vi "RegisterTrends.vi"(8 "error in (no error)":errorcluster, 9 "asset node id":string, 10 "data group":string, 11 "data group map":variant) -> (0 "error out":errorcluster, 3 "data group map":variant)   [LabVIEW 2017, in "ModbusMaster.lvlib"]
uses:
  <vilib>/addons/InsightCM/Devices/Shared/Common/ModbusMaster/ModbusMaster.lvlib
  <vilib>/addons/InsightCM/Devices/Shared/Common/DataEventCreator/controls/Registry_Trend.ctl
  <vilib>/addons/InsightCM/Devices/Shared/Common/DataEventCreator/DataEventCreator.lvlib
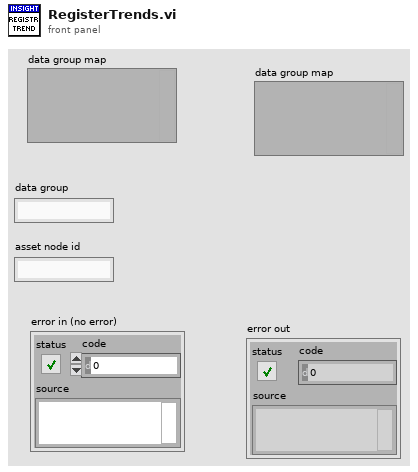
[diagram p1: front panel]
types:
  T1 = typedef "DataEventCreator.lvlib/Registry_Trend.ctl" = cluster{"TrendPointId":string, "DataSetName":string, "HighRate":bool, "Always Send":bool}
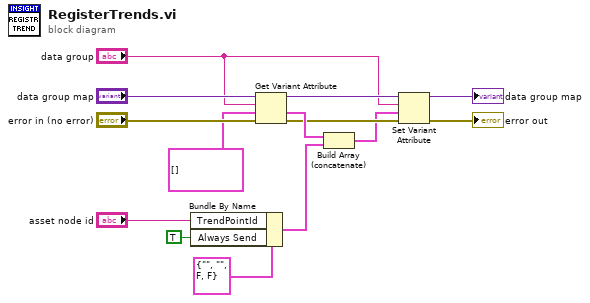
[diagram p0: block diagram]
diagram:
  n1 = Bundle By Name(cluster=T1 {"TrendPointId"="", "DataSetName"="", "HighRate"=FALSE, "Always Send"=FALSE} ("Trend"), "TrendPointId"="asset node id", "Always Send"=TRUE ("HighRate")) -> (w8:T1)
  n2 = Get Variant Attribute(Variant="data group map", name="data group", default value (empty Variant)=T1[] [], error in="error in (no error)") -> (duplicate Variant=w6:variant, value=w9:T1[], error out=w7:errorcluster)  [unwired: 1 out]
  n3 = Build Array (concatenate)(w9, w8) -> (w4:T1[])
  n4 = Set Variant Attribute(Variant=w6, name="data group", value=w4, error in=w7) -> (Variant out=→"data group map":variant, error out=→"error out":errorcluster)  [unwired: 1 out]
